vi "Fdx Write (UDP-CommPort).vi"(8 "error in (no error)":errorcluster, 9 "Data":u8[](array[numeric]) format="%.0x", 10 "UdpHandle in":u32, 11 "InstrumentHandle_port in":u32) -> (0 "error out":errorcluster, 1 "BytesWritten":u32, 2 "UdpHandle out":u32, 3 "InstrumentHandle_port out":u32)   [LabVIEW 2020, in "AIM664LV.lvlib"]
uses:
  AIM664LV.lvlib
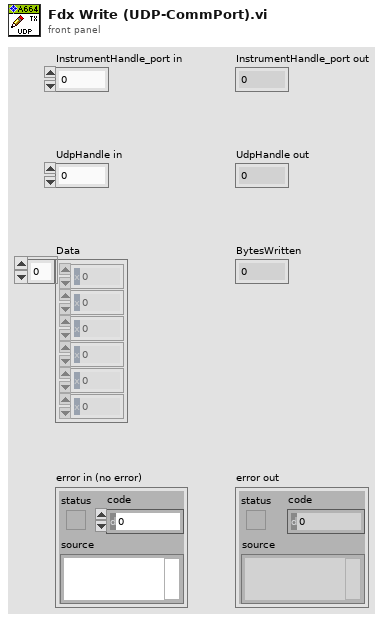
[diagram p1: front panel]
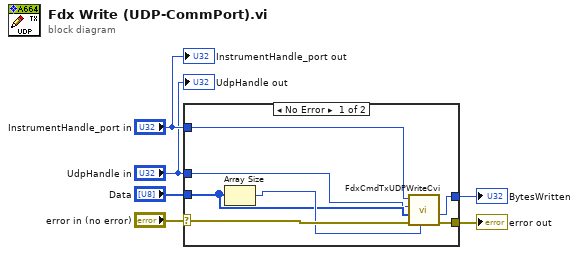
[diagram p0: block diagram]
diagram:
  n1 = case shown="No Error" "error in (no error)" {
    selector: "error in (no error)" -> [w11 w14]
    tunnel: [w13 w14] -> w5
    tunnel: "Data" -> [w8 _]
    tunnel: [w12 _] -> w3
    tunnel: "InstrumentHandle_port in" -> [w10 _]
    tunnel: "UdpHandle in" -> [w7 _]
    frame No Error {
      n2 = Array Size(array=w8) -> (size(s)=w9:i32)
      n3 = call "FdxCmdTxUDPWriteCvi.vi"("ByteCount"=w9, "error in"=w11, "Data"=w8, "UdpHandle"=w7, "InstrumentHandle"=w10) -> ("error out"=w13:errorcluster, "BytesWritten"=w12:u32)  [unwired: 3 in, 2 out]
    }
    frame Error {
    }
  }
  "error out" <- w5
  "BytesWritten" <- w3
  "InstrumentHandle_port out" <- "InstrumentHandle_port in"
  "UdpHandle out" <- "UdpHandle in"
